vi "JKI.Robot.SMO.Main.vi"() -> ()   [LabVIEW 2015]
doc: "JKI State Machine Objects (SMO) 1.0.0.5\nJKI - JKI\nCopyright (c) 2016, JKI"
uses:
  JKI.Robot.SMO.TestUI/JKI.Robot.SMO.APITesterUI.lvclass
  Interfaces/Robot_Interface.Web/Robot_Interface.Web.lvclass
  Interfaces/Robot_Interface.Web/Typedefs/Configuration--Cluster.ctl
  JKI.Robot.SMO.FPGADriver/JKI.Robot.SMO.FPGADriver.lvclass
  JKI.Robot.SMO.FPGADriver/Typedefs/Configuration--Cluster.ctl
  <vilib>/userdefined/Low Color/nirio_resource_lc.ctl
  JKI.Robot.SMO.lvclass
  JKI.Robot.SMO.TestUI/JKI.Robot.SMO.APITesterUI.lvclass/JKI.Robot.SMO.APITesterUI.ctl
  <vilib>/JKI/JKI SMO/SMO/SMO.lvclass
  <vilib>/JKI/JKI SMO/SMO.UI/SMO.UI.lvclass
panel:
  in  "Simulate HW":bool
  out "error out":errorcluster
  in  "Stop":bool
  # "BB9 APP LAUNCHER"
  # "For instructions on how to use the JKI State Machine Objects, examples and video tutorials, visit:\nhttp://jki.net/state-machine-objects/\n\nJKI State Machine Objects™\nhttp://jki.net/state-machine-objects/\nCopyright (C) 2005-2015, JKI <info@jki.net>\nALL RIGHTS RESERVED"
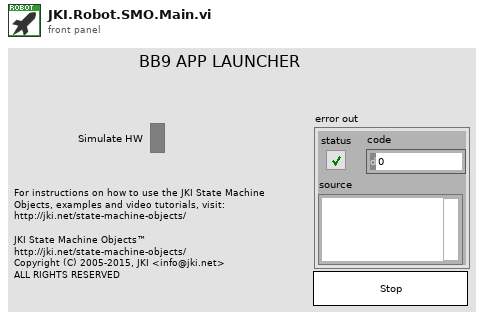
[diagram p1: front panel]
types:
  T1 = typedef "Robot_Interface.Web.lvclass/Configuration--Cluster.ctl" = cluster{"Placeholder":bool, "url":string}
  T2 = typedef "nirio_resource_lc.ctl" = tag
  T3 = typedef "JKI.Robot.SMO.FPGADriver.lvclass/Configuration--Cluster.ctl" = cluster{"RIO Device":T2}
  T4 = cluster{"SMO out":refnum<class "JKI.Robot.SMO.Base.lvclass">}
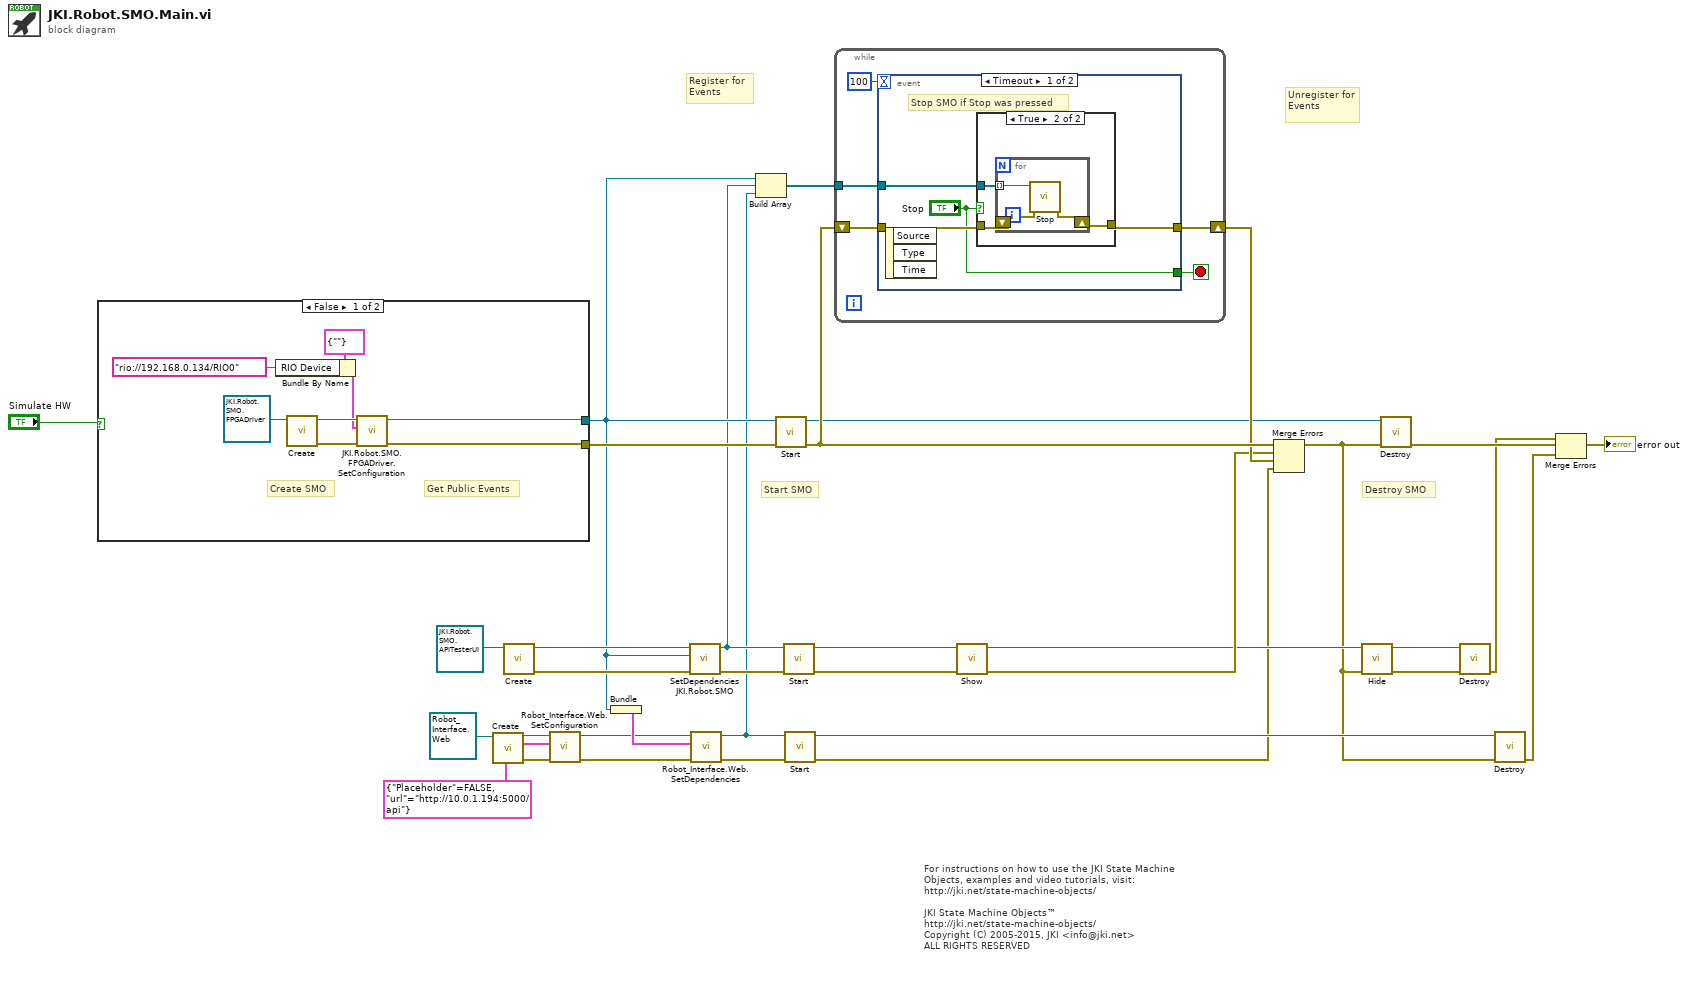
[diagram p0: block diagram]
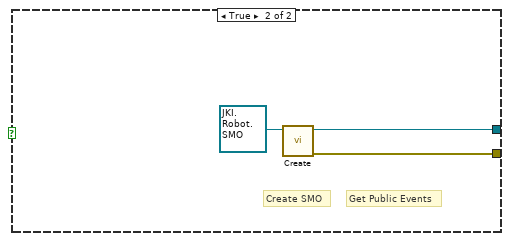
[diagram p2: hidden frame]
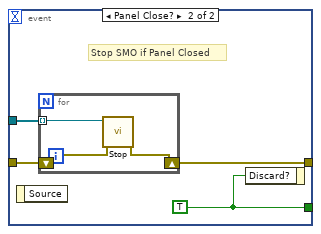
[diagram p4: hidden frame]
diagram:
  # "Start SMO"
  # "Destroy SMO"
  # "For instructions on how to use the JKI State Machine Objects, examples and video tutorials, visit:\nhttp://jki.net/state-machine-objects/\n\nJKI State Machine Objects™\nhttp://jki.net/state-machine-objects/\nCopyright (C) 2005-2015, JKI <info@jki.net>\nALL RIGHTS RESERVED"
  # "Unregister for Events"
  # "Register for Events"
  n1 = case shown="False" "Simulate HW" {
    tunnel: [w39 w43] -> w20
    tunnel: [w35 w45] -> w13
    frame False {
      # "Get Public Events"
      # "Create SMO"
      n2 = Bundle By Name(cluster=T3 {"RIO Device"=""} ("Configuration"), "RIO Device"=T2 "rio://192.168.0.134/RIO0") -> (w37:T3)
      n3 = call <vilib>:"Create.vi"("SMO"=refnum<class "JKI.Robot.SMO.FPGADriver.lvclass"> refnum ("SMO.Template.lvclass")) -> ("error out"=w40:errorcluster, "SMO out"=w41:refnum<class "JKI.Robot.SMO.FPGADriver.lvclass">)  [unwired: 8 in, 1 out]
      n4 = call "JKI.Robot.SMO.FPGADriver.SetConfiguration.vi"("error in (no error)"=w40, "Configuration"=w37, "JKI.Robot.SMO.FPGADriver"=w41) -> ("error out"=w39:errorcluster, "JKI.Robot.SMO.FPGADriver out"=w35:refnum<class "JKI.Robot.SMO.FPGADriver.lvclass">)  [unwired: 7 in]
    }
    frame True {
      # "Get Public Events"
      # "Create SMO"
      n5 = call <vilib>:"Create.vi"("SMO"=refnum<class "JKI.Robot.SMO.lvclass"> refnum ("SMO.Template.lvclass")) -> ("error out"=w43:errorcluster, "SMO out"=w45:refnum<class "JKI.Robot.SMO.lvclass">)  [unwired: 8 in, 1 out]
    }
  }
  n6 = call <vilib>:"Create.vi"("SMO"=refnum<class "Robot_Interface.Web.lvclass"> refnum ("SMO.Template.lvclass")) -> ("error out"=w4:errorcluster, "SMO out"=w5:refnum<class "Robot_Interface.Web.lvclass">)  [unwired: 8 in, 1 out]
  n7 = call <vilib>:"Create.vi"("SMO"=refnum<class "JKI.Robot.SMO.APITesterUI.lvclass"> refnum ("JKI.Robot.SMO.APITesterUI.lvclass")) -> ("error out"=w21:errorcluster, "SMO out"=w22:refnum<class "JKI.Robot.SMO.APITesterUI.lvclass">)  [unwired: 8 in, 1 out]
  n8 = call "Robot_Interface.Web.SetConfiguration.vi"("error in (no error)"=w4, "Configuration"=T1 {"Placeholder"=FALSE, "url"="http://10.0.1.194:5000/api"}, "Robot_Interface.Web"=w5) -> ("error out"=w3:errorcluster, "Robot_Interface.Web out"=w2:refnum<class "Robot_Interface.Web.lvclass">)  [unwired: 7 in]
  n9 = Bundle("SMO out"=w13) -> (w15:T4)  [unwired: 1 in]
  n10 = call "SetDependenciesJKI.Robot.SMO.vi"("error in (no error)"=w21, "JKI.Robot"=w13, "JKI.Robot.SMO.APITesterUI in"=w22) -> ("error out"=w31:errorcluster, "JKI.Robot.SMO.APITesterUI out"=w12:refnum<class "JKI.Robot.SMO.APITesterUI.lvclass">)  [unwired: 7 in]
  n11 = call "Robot_Interface.Web.SetDependencies.vi"("error in (no error)"=w3, "Dependencies"=w15, "Robot_Interface.Web"=w2) -> ("error out"=w14:errorcluster, "Robot_Interface.Web out"=w11:refnum<class "Robot_Interface.Web.lvclass">)  [unwired: 7 in]
  n12 = Build Array(w13, w12, w11) -> (w10:refnum<class "SMO.lvclass">[])
  n13 = call <vilib>:"Start.vi"("error in (no error)"=w20, "SMO"=w13) -> ("error out"=w32:errorcluster, "SMO out"=w19:refnum<class "JKI.Robot.SMO.Base.lvclass">)  [unwired: 8 in]
  n14 = call <vilib>:"Start.vi"("error in (no error)"=w31, "SMO"=w12) -> ("error out"=w28:errorcluster, "SMO out"=w29:refnum<class "JKI.Robot.SMO.APITesterUI.lvclass">)  [unwired: 8 in]
  n15 = call <vilib>:"Start.vi"("error in (no error)"=w14, "SMO"=w11) -> ("error out"=w7:errorcluster, "SMO out"=w8:refnum<class "Robot_Interface.Web.lvclass">)  [unwired: 8 in]
  n16 = while {
    shift-right: [w49] -> w30
    shift-left: w32 -> [w48]
    tunnel: w10 -> [w46]
    stop <- w50 stop-if-true
    n17 = event shown="[0] Timeout" {
      selector: _ -> [_ _]
      dyn-events: _ -> [_ _]
      timeout: 100 -> [_ _]
      tunnel: ["Stop" w63] -> w50
      tunnel: [w54 w65] -> w49
      tunnel: w48 -> [w53 w64]
      tunnel: w46 -> [w51 w62]
      event Timeout {
        # "Stop SMO if Stop was pressed"
        n18 = event-data() -> ()  [unwired: 1 in, 3 out]
        n19 = case shown="True" "Stop" {
          tunnel: [w55 w58] -> w54
          tunnel: w53 -> [w55 w57]
          tunnel: w51 -> [_ w56]
          frame False {
          }
          frame True {
            n20 = for {
              shift-right: [w61] -> w58
              shift-left: w57 -> [w60]
              tunnel: w56 -> [w59] mode=indexing
              n21 = call <vilib>:"Stop.vi"("error in (no error)"=w60, "SMO"=w59) -> ("error out"=w61:errorcluster)  [unwired: 8 in, 1 out]
            }
          }
        }
      }
      event Panel Close? {
        w63 = TRUE ("OK")
        # "Stop SMO if Panel Closed"
        n22 = event-data() -> ()  [unwired: 1 in, 1 out]
        n23 = for {
          shift-right: [w68] -> w65
          shift-left: w64 -> [w67]
          tunnel: w62 -> [w66] mode=indexing
          n24 = call <vilib>:"Stop.vi"("error in (no error)"=w67, "SMO"=w66) -> ("error out"=w68:errorcluster)  [unwired: 8 in, 1 out]
        }
        n25 = event-data("Discard?"=w63) -> ()  [unwired: 1 in, 1 out]
      }
    }
  }
  n26 = call <vilib>:"Show.vi"("error in (no error)"=w28, "SMO.UI"=w29) -> ("error out"=w27:errorcluster, "SMO.UI out"=w26:refnum<class "JKI.Robot.SMO.APITesterUI.lvclass">)  [unwired: 8 in]
  n27 = Merge Errors(w32, w27, w30, w7) -> (w6:errorcluster)
  n28 = call <vilib>:"Hide.vi"("error in (no error)"=w6, "SMO.UI"=w26) -> ("error out"=w24:errorcluster, "SMO.UI out"=w25:refnum<class "JKI.Robot.SMO.APITesterUI.lvclass">)  [unwired: 8 in]
  n29 = call <vilib>:"Destroy.vi"("error in (no error)"=w6, "SMO"=w19) -> ("error out"=w33:errorcluster)  [unwired: 9 in]
  n30 = call <vilib>:"Destroy.vi"("error in (no error)"=w24, "SMO"=w25) -> ("error out"=w18:errorcluster)  [unwired: 9 in]
  n31 = call <vilib>:"Destroy.vi"("error in (no error)"=w6, "SMO"=w8) -> ("error out"=w9:errorcluster)  [unwired: 9 in]
  n32 = Merge Errors(w18, w33, w9) -> (→"error out":errorcluster)
